vi "HDF5_append-dataset-Test5vi.vi"() -> ()   [LabVIEW 2018]
uses:
  <vilib>/addons/h5labview2/file/H5F.lvlib
  <vilib>/addons/h5labview2/file/H5Fmode.ctl
  <vilib>/addons/h5labview2/dataset/H5D.lvlib
  HDF5/HDF5_ToneInfoClust.ctl
  <vilib>/addons/h5labview2/dataset/H5Dwrite.llb/H5Dwrite.xnode
  <vilib>/addons/h5labview2/space/H5S.lvlib
  <vilib>/addons/h5labview2/base/H5Equery.vi
  HDF5/lib_path_mod_20200519.vi
  <vilib>/addons/h5labview2/dataset/H5Dread.llb/H5Dread.xnode
  <vilib>/addons/h5labview2/base/hid_t_renamed.ctl
panel:
  out "Tone2":T1[](array[typedef])
  out "Tone1":T1[](array[typedef])
  in  "data":i32[][](array[numeric])=[[0, 1, 2, 3, 4], [5, 6, 7, 8, 9]]
  out "ms/append":dbl
  out "timer (ms)":u32
  out "progress":i32(slide)=9999 scale=0.0..10000.0
  in  "repetitions":i32=10
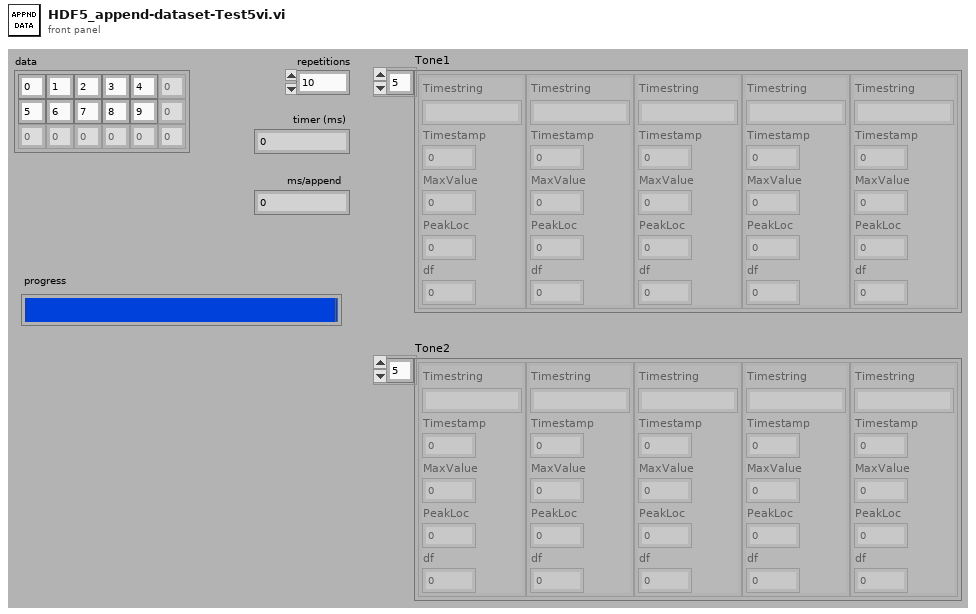
[diagram p1: front panel]
types:
  T1 = typedef "HDF5_ToneInfoClust.ctl" = cluster{"Timestring":string, "Timestamp":dbl, "MaxValue":dbl, "PeakLoc":dbl, "df":dbl}
  T2 = typedef "H5F.lvlib/H5Fmode.ctl" = enum16{"read-only", "read-write", "overwrite", "create new", "open or create"}
  T3 = typedef "HDF5_ToneInfoClust.ctl" = cluster{"Timestring":string, "Timestamp":timestamp, "MaxValue":dbl, "PeakLoc":dbl, "df":dbl}
  T4 = typedef "hid_t.ctl" = i32
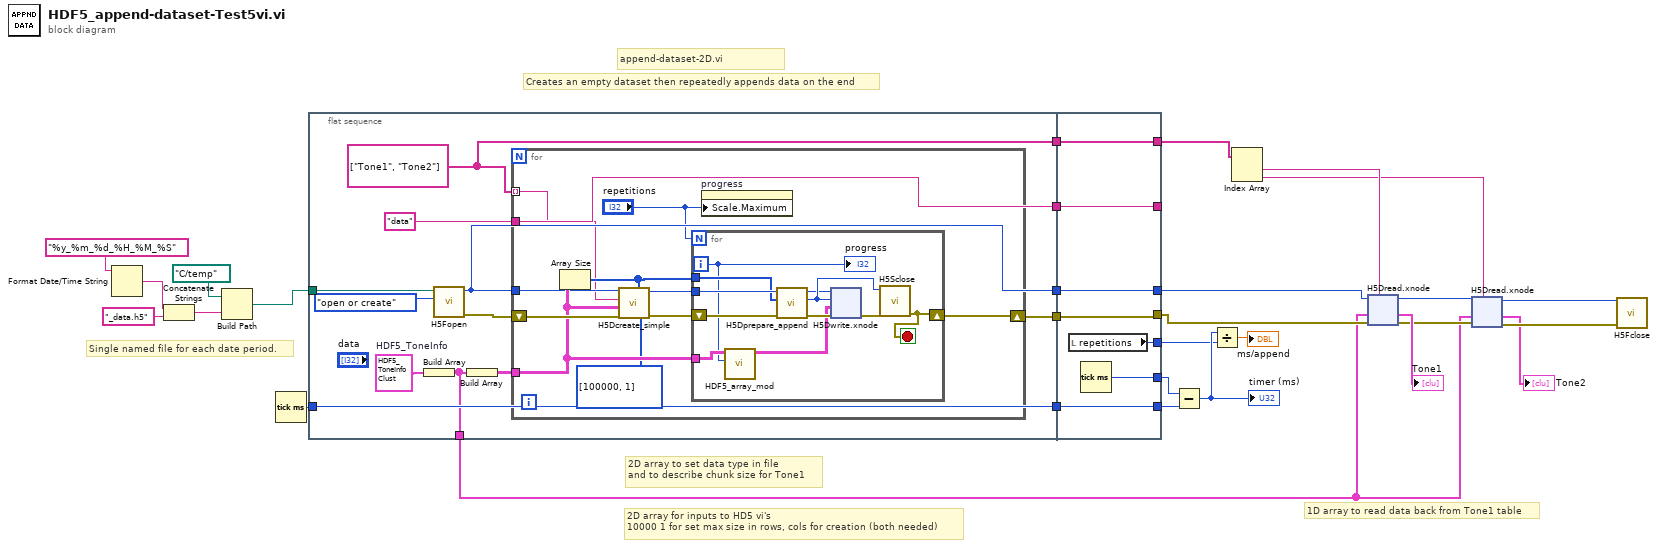
[diagram p0: block diagram]
diagram:
  # "2D array to set data type in file\nand to describe chunk size for Tone1"
  # "1D array to read data back from Tone1 table"
  # "2D array for inputs to HD5 vi's\n10000 1 for set max size in rows, cols for creation (both needed)"
  # "Single named file for each date period."
  # "Creates an empty dataset then repeatedly appends data on the end"
  # "append-dataset-2D.vi"
  n1 = Format Date/Time String(time format string (%c)="%y_%m_%d_%H_%M_%S") -> (date/time string=w19:string)  [unwired: 2 in]
  n2 = Concatenate Strings(w19, "_data.h5" ("string")) -> (w21:string)
  n3 = Build Path(base path=path "C:/temp", name or relative path=w21) -> (appended path=w17:path)
  n4 = Tick Count (ms)() -> (millisecond timer value=w29:u32)
  n5 = flat-sequence {
    tunnel: w29 -> [w38]
    tunnel: [w38] -> w28
    tunnel: w17 -> [w37]
    tunnel: [w34] -> w15
    tunnel: [w33] -> w14
    tunnel: [w32] -> w2
    tunnel: [w31] -> w12
    tunnel: [w30] -> w10
    tunnel: w28 -> [w86]
    tunnel: [w87] -> w27
    tunnel: [w86] -> w26
    tunnel: [w85] -> w24
    tunnel: [w84] -> w16
    tunnel: w15 -> [w84]
    tunnel: [w83] -> _
    tunnel: w14 -> [w83]
    tunnel: [w82] -> w11
    tunnel: w12 -> [w82]
    tunnel: w10 -> [w81]
    tunnel: [w81] -> w8
    frame #0 {
      w30 = string[] ["Tone1", "Tone2"]
      w36 = T3 {"Timestring"="Timestamp string goes here", "Timestamp"=timestamp(0 s since 1904-01-01), "MaxValue"=0.0, "PeakLoc"=0.0, "df"=0.0}  # HDF5_ToneInfo
      w33 = "data" ("name")
      n6 = Build Array(w36) -> (w32:T3[])
      n7 = call <vilib>:"H5Fopen.vi"("mode (read-only)"=H5Fmode."open or create" ("mode"), "path"=w37) -> ("error out"=w39:errorcluster, "ref out"=w34:T4)  [unwired: 8 in]
      n8 = Build Array(w32) -> (w35:T3[][])
      n9 = for {
        tunnel: w35 -> [w46]
        tunnel: w34 -> [w44]
        tunnel: w33 -> [_]
        shift-right: [w43] -> w31
        shift-left: w39 -> [w48]
        tunnel: w30 -> [w42] mode=indexing
        n10 = Array Size(array=w46) -> (size(s)=w45:i32[])
        n11 = call <vilib>:"H5Dcreate_simple.vi"("max size"=u64[] [100000, 1], "chunk size"=w45, "error in (no error)"=w48, "type in"=w46, "name"=w42, "ref in"=w44) -> ("error out"=w49:errorcluster, "dset out"=w50:T4)  [unwired: 4 in]
        n12 = for {
          N: "repetitions" -> [_]
          shift-right: [w57] -> w43
          shift-left: w49 -> [w58]
          tunnel: w45 -> [w59]
          tunnel: w50 -> [w60]
          tunnel: w46 -> [w53]
          i -> [w51]
          stop <- w57 stop-if-true
          n13 = call "HDF5_array_mod.vi"("delta"=w51, "Array in"=w53) -> ("Array out"=w52:T1[][])  [unwired: 9 in]
          n14 = call <vilib>:"H5Dprepare_append.vi"("error in (no error)"=w58, "append dims"=w59, "dset in"=w60) -> ("error out"=w61:errorcluster, "space out"=w55:T4, "dset out"=w54:T4)  [unwired: 5 in, 1 out]
          n15 = xnode "H5Dwrite.xnode"("error in (no error)"=w61, "data"=w52, "file space"=w55, "ref in"=w54) -> ("error out"=w56:errorcluster)  [unwired: 3 in, 2 out]
          n16 = call <vilib>:"H5Sclose.vi"("error in (no error)"=w56, "space in"=w55) -> ("error out"=w57:errorcluster)  [unwired: 9 in]
          "progress" <- w51
        }
        n17 = property on="progress" class="Slide (strict)"("Scale.Maximum"="repetitions") -> ()  [unwired: 2 in, 2 out]
      }
    }
    frame #1 {
      n18 = local read "repetitions"() -> (w85:i32)
      n19 = Tick Count (ms)() -> (millisecond timer value=w87:u32)
    }
  }
  n20 = Subtract(x=w27, y=w26) -> (x-y=w25:u32)
  "timer (ms)" <- w25
  n21 = Divide(x=w25, y=w24) -> (x/y=→"ms/append":dbl)
  n22 = Index Array(array=w8) -> (element #1=w7:string, element #2=w6:string)  [unwired: 2 in]
  n23 = xnode "H5Dread.xnode"("dataset name (this)"=w7, "error in (no error)"=w11, "default"=w2, "ref in"=w16) -> ("error out"=w5:errorcluster, "data"=→"Tone1":T3[], "ref out"=w9:i32)  [unwired: 2 in, 1 out]
  n24 = xnode "H5Dread.xnode"("dataset name (this)"=w6, "error in (no error)"=w5, "default"=w2, "ref in"=w9) -> ("error out"=w3:errorcluster, "data"=→"Tone2":T3[], "ref out"=w4:i32)  [unwired: 2 in, 1 out]
  n25 = call <vilib>:"H5Fclose.vi"("error in (no error)"=w3, "ref"=w4) -> ()  [unwired: 9 in, 1 out]
